vi "SetSweepStep.vi"(8 "error in (no error)":errorcluster, 10 "TX Freq Step Size":dbl format="%.2f") -> (0 "error out":errorcluster)   [LabVIEW 2011]
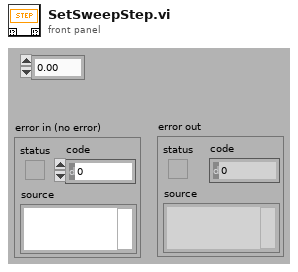
[diagram p1: front panel]
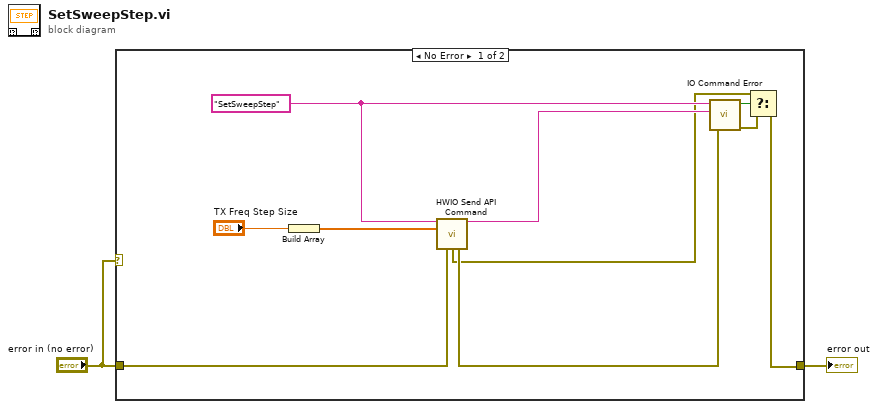
[diagram p0: block diagram]
diagram:
  n1 = case shown="No Error" "error in (no error)" {
    tunnel: "error in (no error)" -> [w12 w13]
    tunnel: [w6 w13] -> w2
    frame No Error {
      w10 = "SetSweepStep"
      n2 = Build Array("TX Freq Step Size") -> (w3:dbl[])
      n3 = call "HWIO Send API Command.vi"("Action"=w10, "Double"=w3, "error in (no error)"=w12) -> ("Action out"=w9:string, "HWError"=w5:errorcluster, "error out"=w11:errorcluster)  [unwired: 5 in, 5 out]
      n4 = call "IO Command Error.vi"("error in (no error)"=w11, "Command Returned (\"\")"=w9, "Command Sent (\"\")"=w10) -> ("error out"=w7:errorcluster, "HW ERR?"=w8:bool)  [unwired: 3 out]
      n5 = Select(t=w5, s=w8, f=w7) -> (s? t:f=w6:errorcluster)
    }
    frame Error {
    }
  }
  "error out" <- w2
